vi "LaserQuantum_Device.vi"(7 "Device-specific in":variant, 8 "error in (no error)":errorcluster, 10 "Position in":dbl[](array[numeric]), 11 "Operation":T2(ring)) -> (0 "error out":errorcluster, 1 "Device properties":cluster{"Axes":string[], "Tolerance":dbl[][]}, 2 "Position out":dbl[](array[numeric]), 3 "Status":T1, 5 "Device-specific out":variant)   [LabVIEW 2018]
uses:
  <vilib>/Instr/_visa.llb/VISA Open Access Mode.ctl
  <vilib>/Instr/_visa.llb/VISA Configure Serial Port (Instr).vi
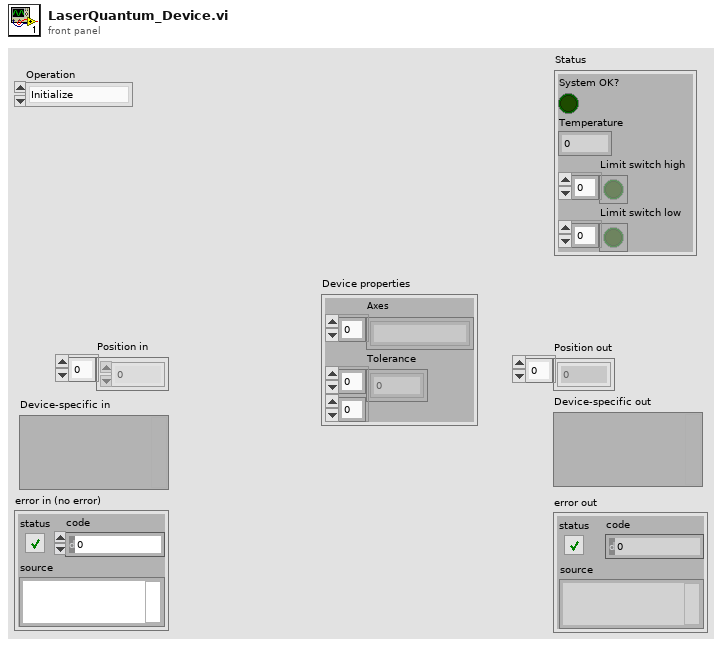
[diagram p1: front panel]
types:
  T1 = cluster{"System OK?":bool, "Temperature":dbl, "Limit switch high":bool[], "Limit switch low":bool[]}
  T2 = enum16{"Initialize", "Shut down", "Set position", "Get position", "Get status", "Other settings"}
  T3 = cluster{"COM port":refnum<visa-resource-name>, "Timeout":u32}
  T4 = typedef "VISA Open Access Mode.ctl" = u32
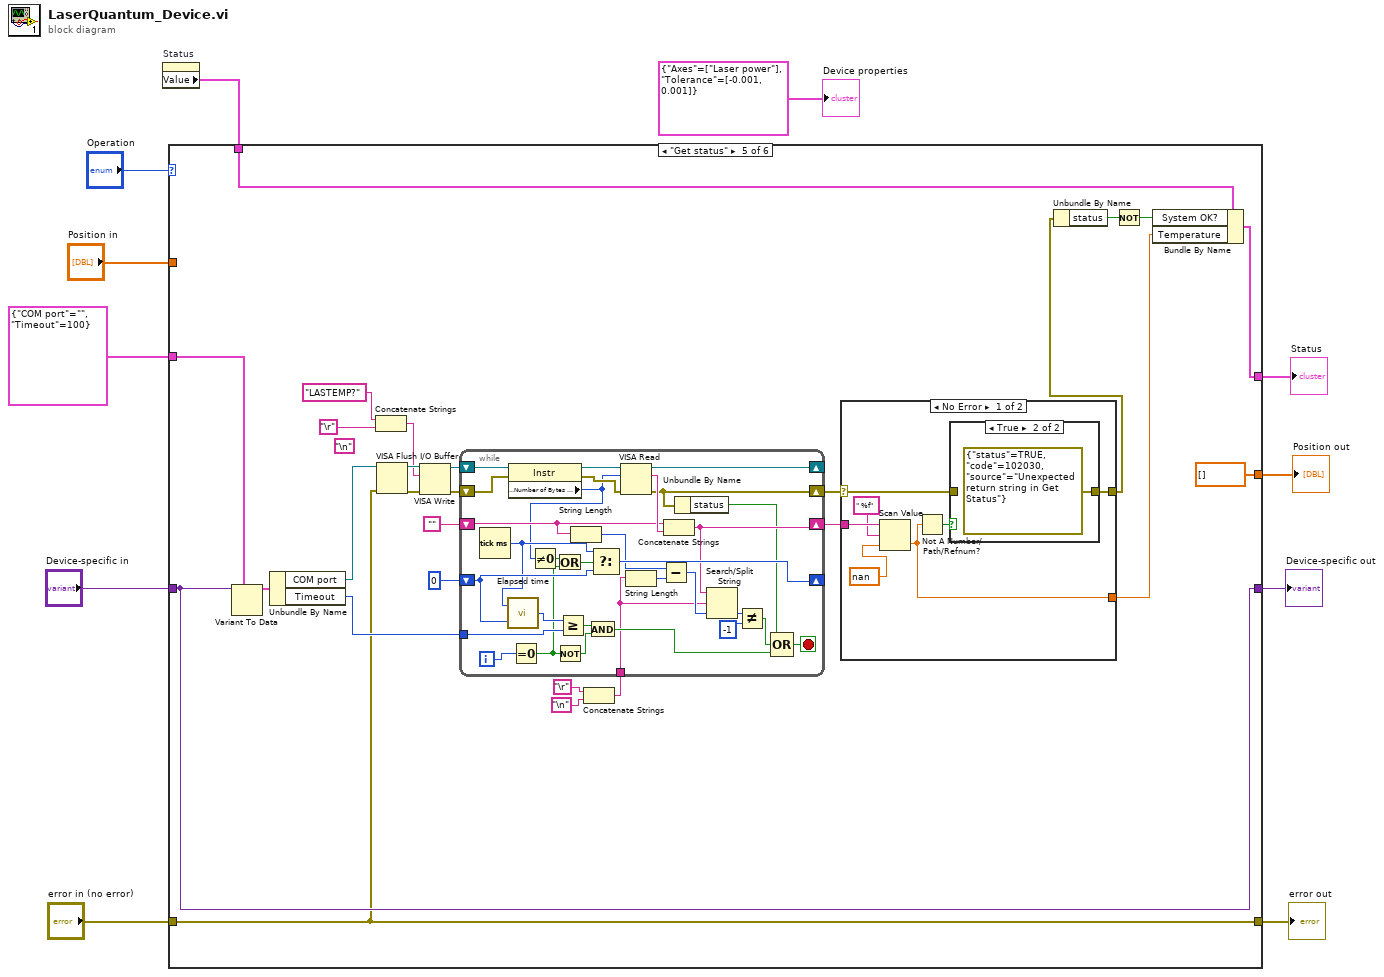
[diagram p0: block diagram]
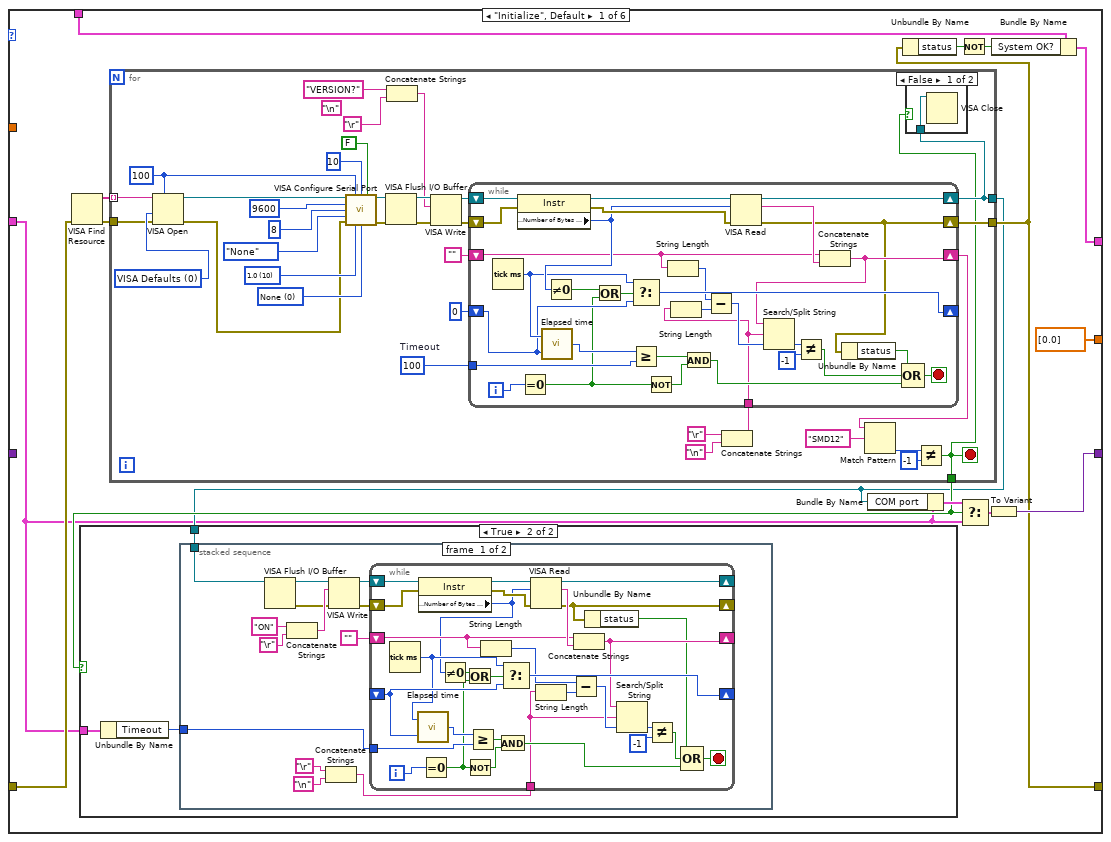
[diagram p2: hidden frame]
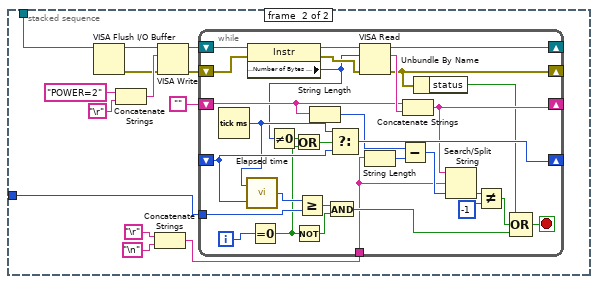
[diagram p4: hidden frame]
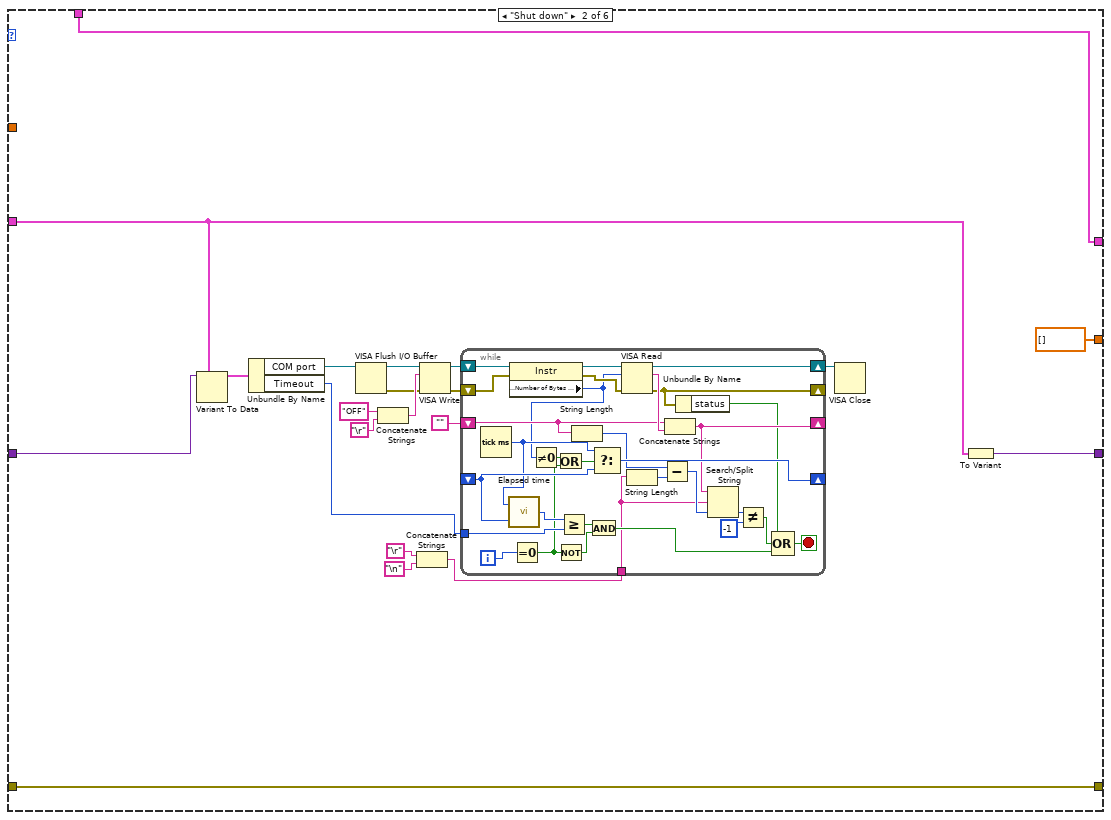
[diagram p6: hidden frame]
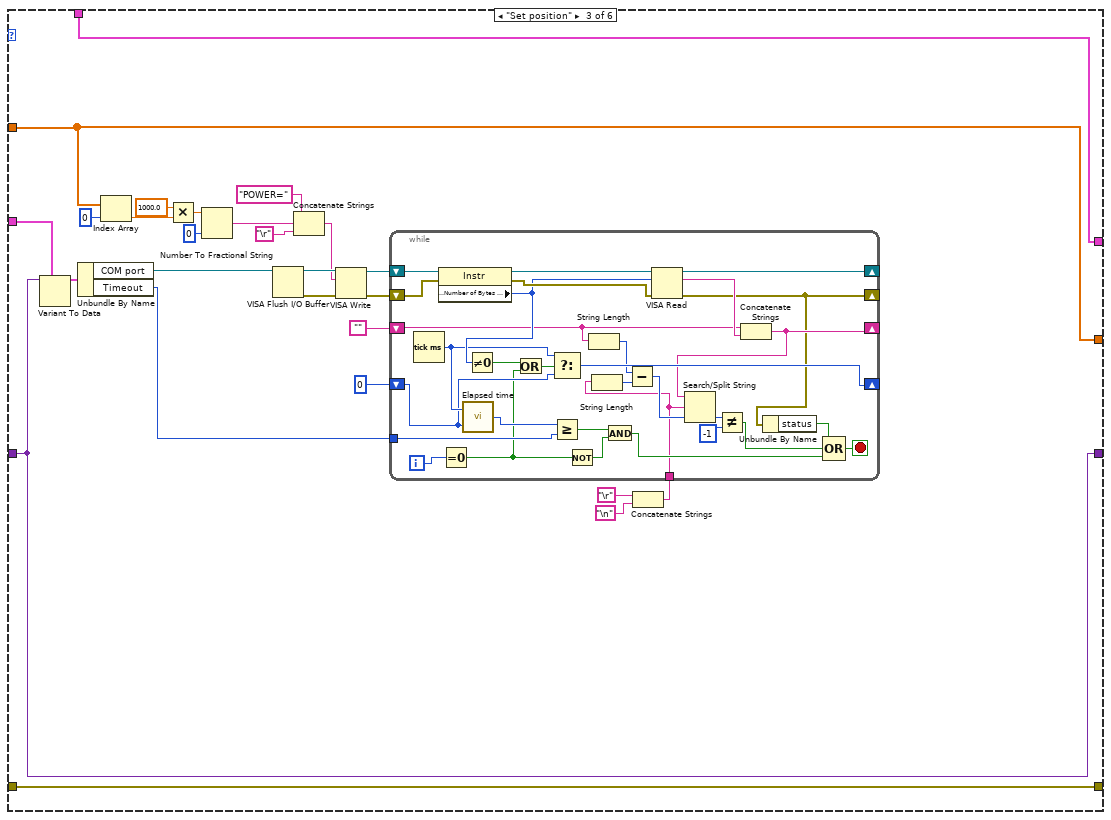
[diagram p7: hidden frame]
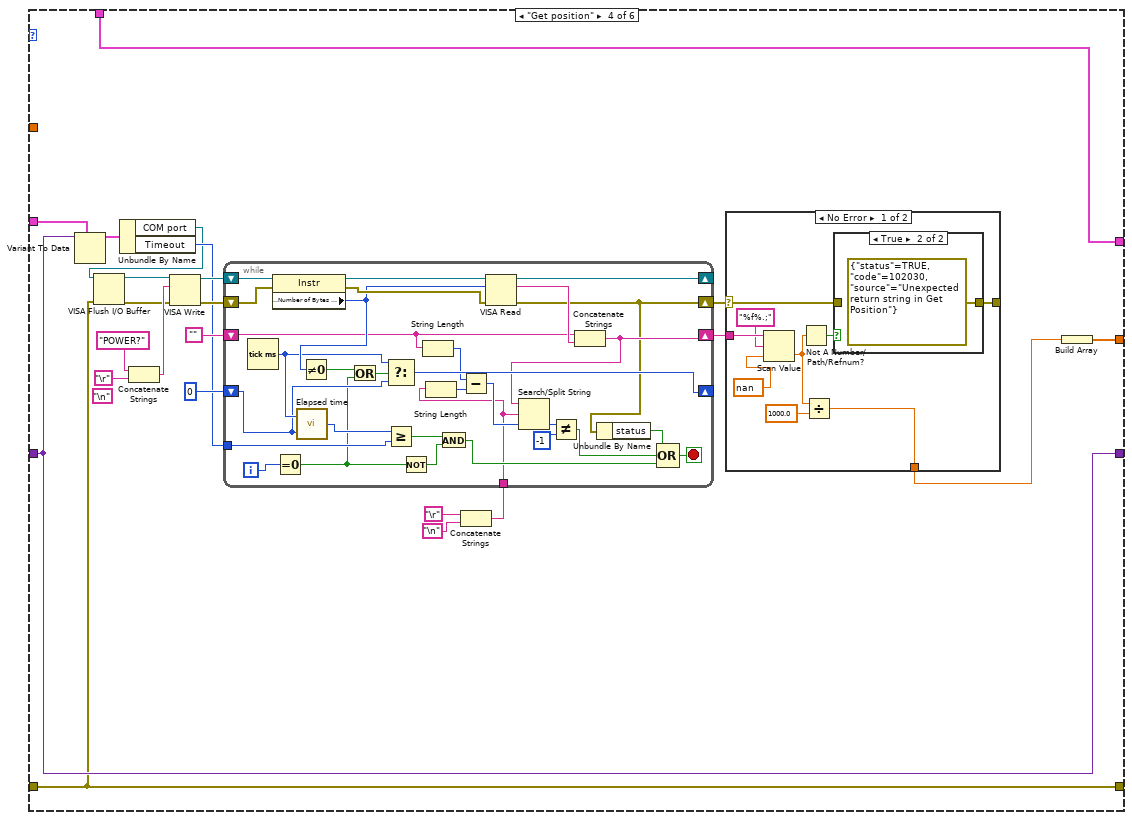
[diagram p8: hidden frame]
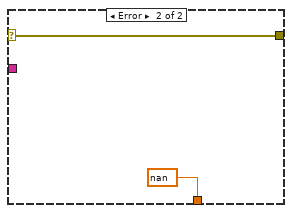
[diagram p10: hidden frame]
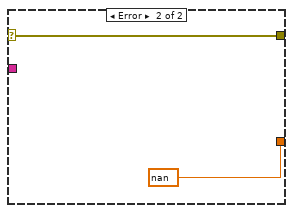
[diagram p12: hidden frame]
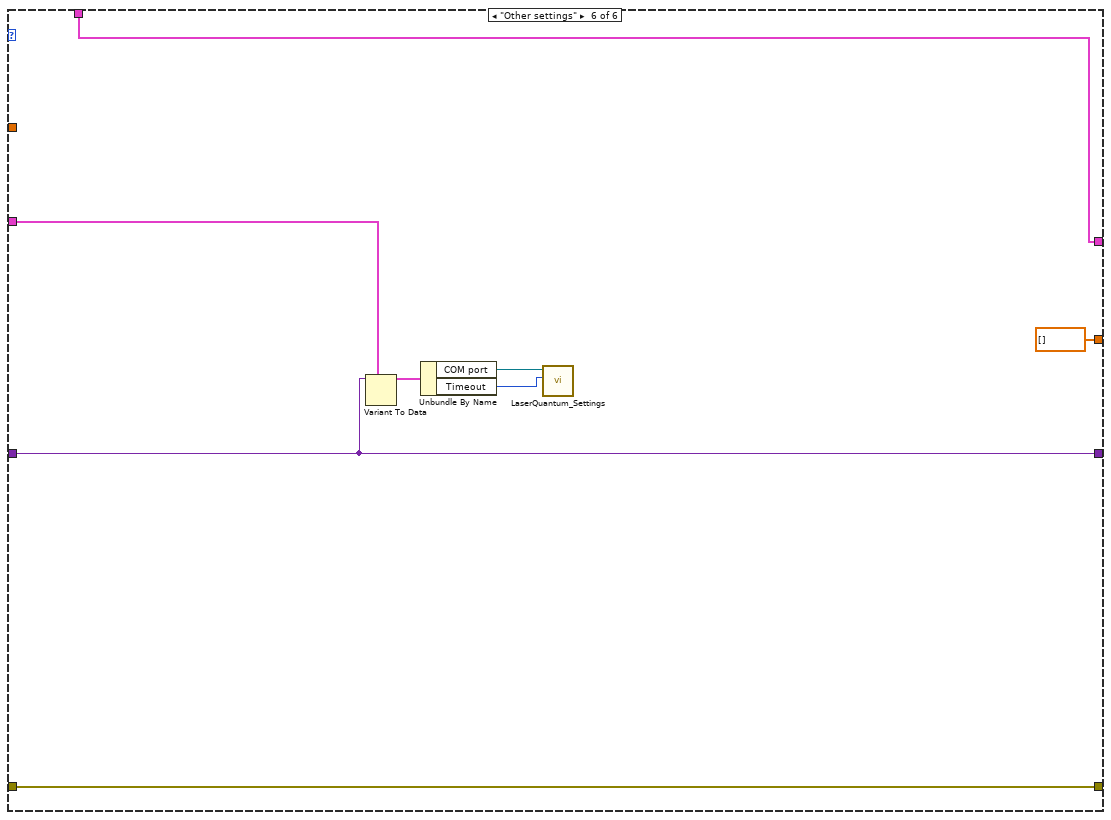
[diagram p13: hidden frame]
diagram:
  n1 = property on="Status" class="Clust (strict)"() -> ("Value"=w10:T1)  [unwired: 2 in, 2 out]
  n2 = case shown="\"Get status\"" "Operation" {
    tunnel: "Position in" -> [_ _ w248 _ _ _]
    tunnel: w10 -> [w26 w205 w262 w316 w387 w437]
    tunnel: [w25 w205 w262 w316 w386 w437] -> w9
    tunnel: "Device-specific in" -> [_ w202 w253 w302 w373 w433]
    tunnel: [dbl[] [0.0] ("Position in") dbl[] [] ("Position in") w248 w303 dbl[] [] ("Position in") dbl[] [] ("Position in")] -> w6
    tunnel: [w20 w199 w253 w302 w373 w433] -> w5
    tunnel: [w17 w204 w261 w294 w364 w436] -> w4
    tunnel: "error in (no error)" -> [w18 w204 w261 w294 w364 w436]
    tunnel: T3 {"COM port"="", "Timeout"=100} -> [w12 w200 w252 w301 w372 w434]
    frame "Initialize", Default {
      n3 = VISA Find Resource(8:w18) -> (0:w19:errorcluster, 3:w23:string[])  [unwired: 2 in, 1 out]
      n4 = for {
        tunnel: w23 -> [w142] mode=indexing
        tunnel: [w123] -> w13
        tunnel: [w122] -> w14
        tunnel: w19 -> [w125]
        tunnel: [w124] -> w17
        stop <- w122 stop-if-true
        w133 = u32 100  # Timeout
        (unwired) "\n"
        w143 = u32 100 ("timeout (10sec)")
        w145 = T4 0 items=["VISA Defaults"=0, "Exclusive Lock"=1, "Load Configured Settings"=4] ("Access Mode")
        w147 = u16 0 items=["None", "XON/XOFF", "RTS/CTS", "XON/XOFF & RTS/CTS", "DTR/DSR", "XON/XOFF & DTR/DSR"] ("flow control (0:none)")
        w148 = u16 10 items=["1.0"=10, "1.5"=15, "2.0"=20] ("stop bits (10: 1 bit)")
        n5 = VISA Open(timeout (0)=w143, access mode=w145, error in (no error)=w125, VISA resource name=w142) -> (VISA resource name=w146:refnum<visa-resource-name>, error out=w144:errorcluster)  [unwired: 1 in]
        n6 = call-poly "VISA Configure Serial Port"("VISA resource name"=w146, "timeout (10sec)"=w143, "termination char\n(0xA = '\\n' = LF)"=u8 10 ("termination char\n(0xA = '\\n' = LF)"), "Enable Termination\nChar (T)"=FALSE ("Enable Termination\nChar (T)"), "baud rate (9600)"=u32 9600, "data bits (8)"=u16 8, "parity (0:none)"=enum16{"None", "Odd", "Even", "Mark", "Space"}."None", "error in (no error)"=w144, "stop bits (10: 1 bit)"=w148, "flow control (0:none)"=w147) -> ("VISA resource name out"=w130:refnum<visa-resource-name>, "error out"=w131:errorcluster)  [unwired: 4 in]
        n7 = VISA Flush I/O Buffer(VISA resource name=w130, error in (no error)=w131) -> (VISA resource name out=w141:refnum<visa-resource-name>, error out=w139:errorcluster)  [unwired: 1 in]
        n8 = Concatenate Strings("VERSION?", "\r") -> (w140:string)
        n9 = VISA Write(VISA resource name=w141, write buffer=w140, error in (no error)=w139) -> (VISA resource name out=w138:refnum<visa-resource-name>, error out=w137:errorcluster)  [unwired: 1 out]
        n10 = Concatenate Strings("\r", "\n") -> (w132:string)
        n11 = while {
          shift-right: [w180] -> w123
          shift-left: w138 -> [w184]
          shift-right: [w154] -> w124
          shift-left: w137 -> [w183]
          shift-right: [w161] -> w129
          shift-left: "" -> [w160]
          shift-right: [w169] -> _
          shift-left: u32 0 -> [w166]
          tunnel: w133 -> [w167]
          tunnel: w132 -> [w155]
          i -> [w172]
          stop <- w179 stop-if-true
          n12 = Tick Count (ms)() -> (millisecond timer value=w170:u32)
          n13 = property class="Instr"(reference=w184, error in=w183) -> (reference out=w182:refnum<visa-resource-name>, error out=w181:errorcluster, "Serial Settings:Number of Bytes at Serial Port"=w174:u32)
          n14 = Equal To 0?(x=w172) -> (x = 0?=w162:bool)
          n15 = call "Elapsed time.vi"("Start time (ms)"=w166, "Current time (ms)"=w170) -> ("Elapsed time"=w168:u32)
          n16 = Not Equal To 0?(x=w174) -> (x != 0?=w173:bool)
          n17 = Or(x=w173, y=w162) -> (x .or. y?=w171:bool)
          n18 = Select(t=w170, s=w171, f=w166) -> (s? t:f=w169:u32)
          n19 = Greater Or Equal?(x=w168, y=w167) -> (x >= y?=w164:bool)
          n20 = Not(x=w162) -> (.not. x?=w163:bool)
          n21 = String Length(string=w160) -> (length=w158:i32)
          n22 = String Length(string=w155) -> (length=w159:i32)
          n23 = And(x=w164, y=w163) -> (x .and. y?=w165:bool)
          n24 = Subtract(x=w158, y=w159) -> (x-y=w157:i32)
          n25 = VISA Read(VISA resource name=w182, byte count=w174, error in (no error)=w181) -> (VISA resource name out=w180:refnum<visa-resource-name>, read buffer=w178:string, error out=w154:errorcluster)  [unwired: 1 out]
          n26 = Concatenate Strings(w160, w178) -> (w161:string)
          n27 = Search/Split String(string=w161, search string/char (-)=w155, offset (0)=w157) -> (offset of match=w177:i32)  [unwired: 2 out]
          n28 = Not Equal?(x=w177, y=-1) -> (x != y?=w175:bool)
          n29 = Unbundle By Name(w154) -> ("status"=w156:bool)
          n30 = Compound Arithmetic op=OR(w156, w175, w165) -> (w179:bool)
        }
        n31 = Match Pattern(string=w129, regular expression="SMD12" ("y")) -> (offset past match=w127:i32)  [unwired: 1 in, 3 out]
        n32 = Not Equal?(x=w127, y=-1) -> (x != y?=w122:bool)
        n33 = case shown="False" w122 {
          tunnel: w123 -> [w153 _]
          frame False {
            n34 = VISA Close(VISA resource name=w153) -> ()  [unwired: 1 in, 1 out]
          }
          frame True {
          }
        }
      }
      n35 = case shown="True" w14 {
        tunnel: w12 -> [_ w29]
        tunnel: w13 -> [_ w27]
        frame False {
        }
        frame True {
          n36 = Unbundle By Name(w29) -> ("Timeout"=w28:u32)
          n37 = stacked-sequence {
            tunnel: w28 -> [w39 w83]
            tunnel: w27 -> [w30 w74]
            frame #0 {
              n38 = VISA Flush I/O Buffer(VISA resource name=w30) -> (VISA resource name out=w36:refnum<visa-resource-name>, error out=w34:errorcluster)  [unwired: 2 in]
              n39 = Concatenate Strings("ON", "\r") -> (w35:string)
              n40 = Concatenate Strings("\r", "\n") -> (w42:string)
              n41 = VISA Write(VISA resource name=w36, write buffer=w35, error in (no error)=w34) -> (VISA resource name out=w33:refnum<visa-resource-name>, error out=w32:errorcluster)  [unwired: 1 out]
              n42 = while {
                shift-right: [w69] -> _
                shift-left: w33 -> [w73]
                shift-right: [w45] -> _
                shift-left: w32 -> [w72]
                shift-right: [w52] -> _
                shift-left: "" -> [w51]
                shift-right: [w60] -> _
                shift-left: _ -> [w57]
                tunnel: w39 -> [w58]
                tunnel: w42 -> [w46]
                i -> [w62]
                stop <- w68 stop-if-true
                n43 = Tick Count (ms)() -> (millisecond timer value=w44:u32)
                n44 = call "Elapsed time.vi"("Start time (ms)"=w57, "Current time (ms)"=w44) -> ("Elapsed time"=w59:u32)
                n45 = property class="Instr"(reference=w73, error in=w72) -> (reference out=w71:refnum<visa-resource-name>, error out=w70:errorcluster, "Serial Settings:Number of Bytes at Serial Port"=w43:u32)
                n46 = Equal To 0?(x=w62) -> (x = 0?=w53:bool)
                n47 = Not Equal To 0?(x=w43) -> (x != 0?=w63:bool)
                n48 = Or(x=w63, y=w53) -> (x .or. y?=w61:bool)
                n49 = Not(x=w53) -> (.not. x?=w54:bool)
                n50 = Greater Or Equal?(x=w59, y=w58) -> (x >= y?=w55:bool)
                n51 = String Length(string=w51) -> (length=w49:i32)
                n52 = And(x=w55, y=w54) -> (x .and. y?=w56:bool)
                n53 = Select(t=w44, s=w61, f=w57) -> (s? t:f=w60:u32)
                n54 = VISA Read(VISA resource name=w71, byte count=w43, error in (no error)=w70) -> (VISA resource name out=w69:refnum<visa-resource-name>, read buffer=w67:string, error out=w45:errorcluster)  [unwired: 1 out]
                n55 = String Length(string=w46) -> (length=w50:i32)
                n56 = Subtract(x=w49, y=w50) -> (x-y=w48:i32)
                n57 = Concatenate Strings(w51, w67) -> (w52:string)
                n58 = Unbundle By Name(w45) -> ("status"=w47:bool)
                n59 = Search/Split String(string=w52, search string/char (-)=w46, offset (0)=w48) -> (offset of match=w66:i32)  [unwired: 2 out]
                n60 = Not Equal?(x=w66, y=-1) -> (x != y?=w64:bool)
                n61 = Compound Arithmetic op=OR(w47, w64, w56) -> (w68:bool)
              }
            }
            frame #1 {
              n62 = VISA Flush I/O Buffer(VISA resource name=w74) -> (VISA resource name out=w80:refnum<visa-resource-name>, error out=w78:errorcluster)  [unwired: 2 in]
              n63 = Concatenate Strings("POWER=2", "\r") -> (w79:string)
              n64 = Concatenate Strings("\r", "\n") -> (w86:string)
              n65 = VISA Write(VISA resource name=w80, write buffer=w79, error in (no error)=w78) -> (VISA resource name out=w77:refnum<visa-resource-name>, error out=w76:errorcluster)  [unwired: 1 out]
              n66 = while {
                shift-right: [w113] -> _
                shift-left: w77 -> [w117]
                shift-right: [w89] -> _
                shift-left: w76 -> [w116]
                shift-right: [w96] -> _
                shift-left: "" -> [w95]
                shift-right: [w104] -> _
                shift-left: _ -> [w101]
                tunnel: w83 -> [w102]
                tunnel: w86 -> [w90]
                i -> [w106]
                stop <- w112 stop-if-true
                n67 = Tick Count (ms)() -> (millisecond timer value=w88:u32)
                n68 = call "Elapsed time.vi"("Start time (ms)"=w101, "Current time (ms)"=w88) -> ("Elapsed time"=w103:u32)
                n69 = property class="Instr"(reference=w117, error in=w116) -> (reference out=w115:refnum<visa-resource-name>, error out=w114:errorcluster, "Serial Settings:Number of Bytes at Serial Port"=w87:u32)
                n70 = Equal To 0?(x=w106) -> (x = 0?=w97:bool)
                n71 = Not Equal To 0?(x=w87) -> (x != 0?=w107:bool)
                n72 = Or(x=w107, y=w97) -> (x .or. y?=w105:bool)
                n73 = Not(x=w97) -> (.not. x?=w98:bool)
                n74 = Greater Or Equal?(x=w103, y=w102) -> (x >= y?=w99:bool)
                n75 = String Length(string=w95) -> (length=w93:i32)
                n76 = And(x=w99, y=w98) -> (x .and. y?=w100:bool)
                n77 = Select(t=w88, s=w105, f=w101) -> (s? t:f=w104:u32)
                n78 = VISA Read(VISA resource name=w115, byte count=w87, error in (no error)=w114) -> (VISA resource name out=w113:refnum<visa-resource-name>, read buffer=w111:string, error out=w89:errorcluster)  [unwired: 1 out]
                n79 = String Length(string=w90) -> (length=w94:i32)
                n80 = Subtract(x=w93, y=w94) -> (x-y=w92:i32)
                n81 = Concatenate Strings(w95, w111) -> (w96:string)
                n82 = Unbundle By Name(w89) -> ("status"=w91:bool)
                n83 = Search/Split String(string=w96, search string/char (-)=w90, offset (0)=w92) -> (offset of match=w110:i32)  [unwired: 2 out]
                n84 = Not Equal?(x=w110, y=-1) -> (x != y?=w108:bool)
                n85 = Compound Arithmetic op=OR(w91, w108, w100) -> (w112:bool)
              }
            }
          }
        }
      }
      n86 = Bundle By Name(cluster=w12, "COM port"=w13) -> (w22:T3)
      n87 = Unbundle By Name(w17) -> ("status"=w16:bool)
      n88 = Not(x=w16) -> (.not. x?=w15:bool)
      n89 = Select(t=w22, s=w14, f=w12) -> (s? t:f=w21:T3)
      n90 = To Variant(anything=w21) -> (Variant=w20:variant)
      n91 = Bundle By Name(cluster=w26, "System OK?"=w15) -> (w25:T1)
    }
    frame "Shut down" {
      n92 = Variant To Data(type=w200, Variant=w202) -> (data=w201:T3)  [unwired: 1 in, 1 out]
      n93 = Unbundle By Name(w201) -> ("COM port"=w198:refnum<visa-resource-name>, "Timeout"=w196:u32)
      n94 = VISA Flush I/O Buffer(VISA resource name=w198) -> (VISA resource name out=w190:refnum<visa-resource-name>, error out=w188:errorcluster)  [unwired: 2 in]
      n95 = Concatenate Strings("OFF", "\r") -> (w189:string)
      n96 = Concatenate Strings("\r", "\n") -> (w195:string)
      n97 = VISA Write(VISA resource name=w190, write buffer=w189, error in (no error)=w188) -> (VISA resource name out=w187:refnum<visa-resource-name>, error out=w186:errorcluster)  [unwired: 1 out]
      n98 = while {
        shift-right: [w232] -> w197
        shift-left: w187 -> [w236]
        shift-right: [w208] -> _
        shift-left: w186 -> [w235]
        shift-right: [w215] -> _
        shift-left: "" -> [w214]
        shift-right: [w223] -> _
        shift-left: _ -> [w220]
        tunnel: w196 -> [w221]
        tunnel: w195 -> [w209]
        i -> [w225]
        stop <- w231 stop-if-true
        n99 = Tick Count (ms)() -> (millisecond timer value=w207:u32)
        n100 = call "Elapsed time.vi"("Start time (ms)"=w220, "Current time (ms)"=w207) -> ("Elapsed time"=w222:u32)
        n101 = property class="Instr"(reference=w236, error in=w235) -> (reference out=w234:refnum<visa-resource-name>, error out=w233:errorcluster, "Serial Settings:Number of Bytes at Serial Port"=w206:u32)
        n102 = Equal To 0?(x=w225) -> (x = 0?=w216:bool)
        n103 = Not Equal To 0?(x=w206) -> (x != 0?=w226:bool)
        n104 = Or(x=w226, y=w216) -> (x .or. y?=w224:bool)
        n105 = Not(x=w216) -> (.not. x?=w217:bool)
        n106 = Greater Or Equal?(x=w222, y=w221) -> (x >= y?=w218:bool)
        n107 = String Length(string=w214) -> (length=w212:i32)
        n108 = And(x=w218, y=w217) -> (x .and. y?=w219:bool)
        n109 = Select(t=w207, s=w224, f=w220) -> (s? t:f=w223:u32)
        n110 = VISA Read(VISA resource name=w234, byte count=w206, error in (no error)=w233) -> (VISA resource name out=w232:refnum<visa-resource-name>, read buffer=w230:string, error out=w208:errorcluster)  [unwired: 1 out]
        n111 = String Length(string=w209) -> (length=w213:i32)
        n112 = Subtract(x=w212, y=w213) -> (x-y=w211:i32)
        n113 = Concatenate Strings(w214, w230) -> (w215:string)
        n114 = Unbundle By Name(w208) -> ("status"=w210:bool)
        n115 = Search/Split String(string=w215, search string/char (-)=w209, offset (0)=w211) -> (offset of match=w229:i32)  [unwired: 2 out]
        n116 = Not Equal?(x=w229, y=-1) -> (x != y?=w227:bool)
        n117 = Compound Arithmetic op=OR(w210, w227, w219) -> (w231:bool)
      }
      n118 = VISA Close(VISA resource name=w197) -> ()  [unwired: 1 in, 1 out]
      n119 = To Variant(anything=w200) -> (Variant=w199:variant)
    }
    frame "Set position" {
      n120 = Variant To Data(type=w252, Variant=w253) -> (data=w251:T3)  [unwired: 1 in, 1 out]
      n121 = Unbundle By Name(w251) -> ("COM port"=w249:refnum<visa-resource-name>, "Timeout"=w250:u32)
      n122 = Index Array(array=w248, index=0) -> (element=w244:dbl)
      n123 = Multiply(x=1000.0, y=w244) -> (x*y=w241:dbl)
      n124 = Number To Fractional String(number=w241, precision (6)=i16 0) -> (F-format string=w243:string)  [unwired: 2 in]
      n125 = VISA Flush I/O Buffer(VISA resource name=w249) -> (VISA resource name out=w260:refnum<visa-resource-name>, error out=w259:errorcluster)  [unwired: 2 in]
      n126 = Concatenate Strings("POWER=", w243, "\r") -> (w246:string)
      n127 = VISA Write(VISA resource name=w260, write buffer=w246, error in (no error)=w259) -> (VISA resource name out=w258:refnum<visa-resource-name>, error out=w257:errorcluster)  [unwired: 1 out]
      n128 = Concatenate Strings("\r", "\n") -> (w254:string)
      n129 = while {
        shift-right: [w289] -> _
        shift-left: w258 -> [w293]
        shift-right: [w263] -> _
        shift-left: w257 -> [w292]
        shift-right: [w270] -> _
        shift-left: "" -> [w269]
        shift-right: [w278] -> _
        shift-left: u32 0 -> [w275]
        tunnel: w250 -> [w276]
        tunnel: w254 -> [w264]
        i -> [w281]
        stop <- w288 stop-if-true
        n130 = Tick Count (ms)() -> (millisecond timer value=w279:u32)
        n131 = property class="Instr"(reference=w293, error in=w292) -> (reference out=w291:refnum<visa-resource-name>, error out=w290:errorcluster, "Serial Settings:Number of Bytes at Serial Port"=w283:u32)
        n132 = Equal To 0?(x=w281) -> (x = 0?=w271:bool)
        n133 = call "Elapsed time.vi"("Start time (ms)"=w275, "Current time (ms)"=w279) -> ("Elapsed time"=w277:u32)
        n134 = Not Equal To 0?(x=w283) -> (x != 0?=w282:bool)
        n135 = Or(x=w282, y=w271) -> (x .or. y?=w280:bool)
        n136 = Select(t=w279, s=w280, f=w275) -> (s? t:f=w278:u32)
        n137 = Greater Or Equal?(x=w277, y=w276) -> (x >= y?=w273:bool)
        n138 = Not(x=w271) -> (.not. x?=w272:bool)
        n139 = String Length(string=w269) -> (length=w267:i32)
        n140 = String Length(string=w264) -> (length=w268:i32)
        n141 = And(x=w273, y=w272) -> (x .and. y?=w274:bool)
        n142 = Subtract(x=w267, y=w268) -> (x-y=w266:i32)
        n143 = VISA Read(VISA resource name=w291, byte count=w283, error in (no error)=w290) -> (VISA resource name out=w289:refnum<visa-resource-name>, read buffer=w287:string, error out=w263:errorcluster)  [unwired: 1 out]
        n144 = Concatenate Strings(w269, w287) -> (w270:string)
        n145 = Search/Split String(string=w270, search string/char (-)=w264, offset (0)=w266) -> (offset of match=w286:i32)  [unwired: 2 out]
        n146 = Not Equal?(x=w286, y=-1) -> (x != y?=w284:bool)
        n147 = Unbundle By Name(w263) -> ("status"=w265:bool)
        n148 = Compound Arithmetic op=OR(w265, w284, w274) -> (w288:bool)
      }
    }
    frame "Get position" {
      (unwired) "\n"
      n149 = Variant To Data(type=w301, Variant=w302) -> (data=w300:T3)  [unwired: 1 in, 1 out]
      n150 = Unbundle By Name(w300) -> ("COM port"=w298:refnum<visa-resource-name>, "Timeout"=w299:u32)
      n151 = VISA Flush I/O Buffer(VISA resource name=w298, error in (no error)=w294) -> (VISA resource name out=w315:refnum<visa-resource-name>, error out=w313:errorcluster)  [unwired: 1 in]
      n152 = Concatenate Strings("POWER?", "\r") -> (w314:string)
      n153 = VISA Write(VISA resource name=w315, write buffer=w314, error in (no error)=w313) -> (VISA resource name out=w312:refnum<visa-resource-name>, error out=w311:errorcluster)  [unwired: 1 out]
      n154 = Concatenate Strings("\r", "\n") -> (w305:string)
      n155 = while {
        shift-right: [w356] -> _
        shift-left: w312 -> [w360]
        shift-right: [w330] -> w306
        shift-left: w311 -> [w359]
        shift-right: [w337] -> w307
        shift-left: "" -> [w336]
        shift-right: [w345] -> _
        shift-left: u32 0 -> [w342]
        tunnel: w299 -> [w343]
        tunnel: w305 -> [w331]
        i -> [w348]
        stop <- w355 stop-if-true
        n156 = Tick Count (ms)() -> (millisecond timer value=w346:u32)
        n157 = property class="Instr"(reference=w360, error in=w359) -> (reference out=w358:refnum<visa-resource-name>, error out=w357:errorcluster, "Serial Settings:Number of Bytes at Serial Port"=w350:u32)
        n158 = Equal To 0?(x=w348) -> (x = 0?=w338:bool)
        n159 = call "Elapsed time.vi"("Start time (ms)"=w342, "Current time (ms)"=w346) -> ("Elapsed time"=w344:u32)
        n160 = Not Equal To 0?(x=w350) -> (x != 0?=w349:bool)
        n161 = Or(x=w349, y=w338) -> (x .or. y?=w347:bool)
        n162 = Select(t=w346, s=w347, f=w342) -> (s? t:f=w345:u32)
        n163 = Greater Or Equal?(x=w344, y=w343) -> (x >= y?=w340:bool)
        n164 = Not(x=w338) -> (.not. x?=w339:bool)
        n165 = String Length(string=w336) -> (length=w334:i32)
        n166 = String Length(string=w331) -> (length=w335:i32)
        n167 = And(x=w340, y=w339) -> (x .and. y?=w341:bool)
        n168 = Subtract(x=w334, y=w335) -> (x-y=w333:i32)
        n169 = VISA Read(VISA resource name=w358, byte count=w350, error in (no error)=w357) -> (VISA resource name out=w356:refnum<visa-resource-name>, read buffer=w354:string, error out=w330:errorcluster)  [unwired: 1 out]
        n170 = Concatenate Strings(w336, w354) -> (w337:string)
        n171 = Search/Split String(string=w337, search string/char (-)=w331, offset (0)=w333) -> (offset of match=w353:i32)  [unwired: 2 out]
        n172 = Not Equal?(x=w353, y=-1) -> (x != y?=w351:bool)
        n173 = Unbundle By Name(w330) -> ("status"=w332:bool)
        n174 = Compound Arithmetic op=OR(w332, w351, w341) -> (w355:bool)
      }
      n175 = case shown="No Error" w306 {
        selector: w306 -> [w324 w329]
        tunnel: w307 -> [w322 _]
        tunnel: [w325 w329] -> _
        tunnel: [w319 nan] -> w304
        frame No Error {
          n176 = Scan Value(string=w322, format string="%f%.;", default (0 dbl)=nan ("t")) -> (value=w318:dbl)  [unwired: 1 out]
          n177 = Not A Number/Path/Refnum?(number/path/refnum=w318) -> (NaN/Path/Refnum?=w323:bool)
          n178 = Divide(x=w318, y=1000.0) -> (x/y=w319:dbl)
          n179 = case shown="True" w323 {
            tunnel: [w326 errorcluster {"status"=TRUE, "code"=102030, "source"="Unexpected return string in Get Position"} ("error IO")] -> w325
            tunnel: w324 -> [w326 _]
            frame False {
            }
            frame True {
            }
          }
        }
        frame Error {
        }
      }
      n180 = Build Array(w304) -> (w303:dbl[])
    }
    frame "Get status" {
      (unwired) "\n"
      n181 = Variant To Data(type=w372, Variant=w373) -> (data=w371:T3)  [unwired: 1 in, 1 out]
      n182 = Unbundle By Name(w371) -> ("COM port"=w369:refnum<visa-resource-name>, "Timeout"=w370:u32)
      n183 = Concatenate Strings("LASTEMP?", "\r") -> (w374:string)
      n184 = VISA Flush I/O Buffer(VISA resource name=w369, error in (no error)=w364) -> (VISA resource name out=w384:refnum<visa-resource-name>, error out=w383:errorcluster)  [unwired: 1 in]
      n185 = VISA Write(VISA resource name=w384, write buffer=w374, error in (no error)=w383) -> (VISA resource name out=w382:refnum<visa-resource-name>, error out=w381:errorcluster)  [unwired: 1 out]
      n186 = Concatenate Strings("\r", "\n") -> (w376:string)
      n187 = while {
        shift-right: [w425] -> _
        shift-left: w382 -> [w429]
        shift-right: [w401] -> w367
        shift-left: w381 -> [w428]
        shift-right: [w408] -> w366
        shift-left: "" -> [w407]
        shift-right: [w416] -> _
        shift-left: u32 0 -> [w413]
        tunnel: w370 -> [w414]
        tunnel: w376 -> [w402]
        i -> [w418]
        stop <- w424 stop-if-true
        n188 = Tick Count (ms)() -> (millisecond timer value=w400:u32)
        n189 = call "Elapsed time.vi"("Start time (ms)"=w413, "Current time (ms)"=w400) -> ("Elapsed time"=w415:u32)
        n190 = property class="Instr"(reference=w429, error in=w428) -> (reference out=w427:refnum<visa-resource-name>, error out=w426:errorcluster, "Serial Settings:Number of Bytes at Serial Port"=w399:u32)
        n191 = Equal To 0?(x=w418) -> (x = 0?=w409:bool)
        n192 = Not Equal To 0?(x=w399) -> (x != 0?=w419:bool)
        n193 = Or(x=w419, y=w409) -> (x .or. y?=w417:bool)
        n194 = Not(x=w409) -> (.not. x?=w410:bool)
        n195 = Greater Or Equal?(x=w415, y=w414) -> (x >= y?=w411:bool)
        n196 = String Length(string=w407) -> (length=w405:i32)
        n197 = And(x=w411, y=w410) -> (x .and. y?=w412:bool)
        n198 = Select(t=w400, s=w417, f=w413) -> (s? t:f=w416:u32)
        n199 = VISA Read(VISA resource name=w427, byte count=w399, error in (no error)=w426) -> (VISA resource name out=w425:refnum<visa-resource-name>, read buffer=w423:string, error out=w401:errorcluster)  [unwired: 1 out]
        n200 = String Length(string=w402) -> (length=w406:i32)
        n201 = Subtract(x=w405, y=w406) -> (x-y=w404:i32)
        n202 = Concatenate Strings(w407, w423) -> (w408:string)
        n203 = Unbundle By Name(w401) -> ("status"=w403:bool)
        n204 = Search/Split String(string=w408, search string/char (-)=w402, offset (0)=w404) -> (offset of match=w422:i32)  [unwired: 2 out]
        n205 = Not Equal?(x=w422, y=-1) -> (x != y?=w420:bool)
        n206 = Compound Arithmetic op=OR(w403, w420, w412) -> (w424:bool)
      }
      n207 = case shown="No Error" w367 {
        selector: w367 -> [w393 w398]
        tunnel: w366 -> [w391 _]
        tunnel: [w394 w398] -> w363
        tunnel: [w388 nan] -> w365
        frame No Error {
          n208 = Scan Value(string=w391, format string=" %f", default (0 dbl)=nan ("t")) -> (value=w388:dbl)  [unwired: 1 out]
          n209 = Not A Number/Path/Refnum?(number/path/refnum=w388) -> (NaN/Path/Refnum?=w392:bool)
          n210 = case shown="True" w392 {
            tunnel: [w395 errorcluster {"status"=TRUE, "code"=102030, "source"="Unexpected return string in Get Status"} ("error IO")] -> w394
            tunnel: w393 -> [w395 _]
            frame False {
            }
            frame True {
            }
          }
        }
        frame Error {
        }
      }
      n211 = Unbundle By Name(w363) -> ("status"=w362:bool)
      n212 = Not(x=w362) -> (.not. x?=w361:bool)
      n213 = Bundle By Name(cluster=w387, "System OK?"=w361, "Temperature"=w365) -> (w386:T1)
    }
    frame "Other settings" {
      n214 = Variant To Data(type=w434, Variant=w433) -> (data=w432:T3)  [unwired: 1 in, 1 out]
      n215 = Unbundle By Name(w432) -> ("COM port"=w431:refnum<visa-resource-name>, "Timeout"=w430:u32)
      n216 = call "LaserQuantum_Settings.vi"("Timeout"=w430, "COM port"=w431) -> ()  [unwired: 9 in, 1 out]
    }
  }
  "Status" <- w9
  "Device-specific out" <- w5
  "error out" <- w4
  "Position out" <- w6
  "Device properties" <- cluster{"Axes":string[], "Tolerance":dbl[][]} {"Axes"=["Laser power"], "Tolerance"=[[-0.001, 0.001]]} ("Device properties")
